vi "Fpga-AXI-Stream.vi"() -> ()   [LabVIEW 2017]
uses:
  <vilib>/Platform/TimedLoop/XDataNode/timing_clust.ctl
  <vilib>/Platform/TimedLoop/XDataNode/nitl_modes.ctl
  <vilib>/Platform/TimedLoop/XDataNode/wakeup.ctl
  <vilib>/rvi/Emulation/niFpgaSctlEmulationGetInTimedLoop.vi
  <vilib>/rvi/Emulation/niFpgaEmulationReportErrorSimple.vi
  <vilib>/rvi/Emulation/niFpgaGetClockAttributes.vi
  <vilib>/rvi/Emulation/niFpgaCriticalErrorInLSC.vi
  <vilib>/rvi/interface/RandomDataEmulation/niFpgaRandomDataHandleErrors.vi
  <vilib>/Platform/TimedLoop/XDataNode/XDataNode.xnode
  <vilib>/rvi/DataTransferAndStorage/Container/XNode/niFpgaContainer.xnode
  <vilib>/rvi/interface/RandomDataEmulation/nirviRandomDataFpgaReadWriteTemplate.vi
  <vilib>/Platform/TimedLoop/XDataNode/XDNodeRunTimeDep.lvlib
  <vilib>/rvi/IPIntegrationNode/IPINode_Typedef/niFpgaIPINodeSupportedFamilies.ctl
  <vilib>/rvi/IPIntegrationNode/IPINode_Utilities/niFpgaIPINodeSimCore.vi
  <vilib>/rvi/IPIntegrationNode/IPINode_Xnode/niFpgaIPINode.xnode
  IP_Block_1SimFiles/xsim.dir/d_microblaze_wrapper_top/xsimkD566ABB023B84B7CB0097135CB091ED7.dll
panel:
  in  "sys_reset":bool
  in  "AXI_STR_RXD_tvalid":bool
  in  "AXI_STR_RXD_tlast":bool
  in  "AXI_STR_RXD_tdata":u32
  in  "AXI_STR_TXD_tready":bool
  out "AXI_STR_RXD_tready":bool
  out "AXI_STR_TXD_tvalid":bool
  out "AXI_STR_TXD_tlast":bool
  out "GPIO2_tri_o":u32
  out "AXI_STR_TXD_tdata":u32
  in  "GPIO1_tri_i":u32
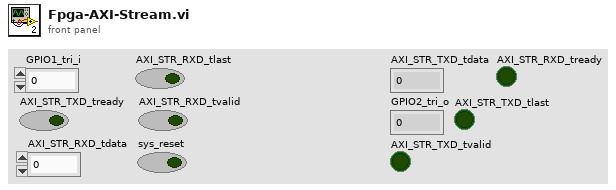
[diagram p1: front panel]
types:
  T1 = typedef "XDNodeRunTimeDep.lvlib/timing_clust.ctl" = cluster{"Expected End [f-1]":u64, "Actual End [f-1]":u64, "Finished Late? [f-1]":bool, "Expected End [i-1]":u64, "Actual End [i-1]":u64, "Finished Late? [i-1]":bool, "Expected Start [i]":u64, "Actual Start [i]":u64, "Expected Start [f]":u64, "Actual Start [f]":u64, "Source Name":string, "Structure Name":string, "Period":i64, "Deadline":i64, "Offset":i64, "Start":i64, "Priority":i32, "Timeout":i32, "Mode":T2, "Wakeup Reason":T3, "Error":errorcluster, "Source Type":string, "Secondary Source Type":string, "Global End Time":u64, "Global Start Time":u64, "Frame Duration":u64, "Iteration Duration":u64, "Assigned CPU":i32, "I/O Scan Engine Mode":u32}
  T2 = typedef "XDNodeRunTimeDep.lvlib/nitl_modes.ctl" = enum32{"No Change", "Process missed periods, maintain original phase", "Discard missed periods, maintain original phase", "Process missed periods, ignore original phase", "Discard missed periods, ignore original phase"}
  T3 = typedef "XDNodeRunTimeDep.lvlib/wakeup.ctl" = enum32{"Normal", "Aborted", "Asynchronous wakeup", "Timing source error", "Timed loop error", "Timeout"}
  T4 = typedef "niFpgaIPINodeSupportedFamilies.ctl" = cluster{"unlimited?":bool, "supported targets":string[]}
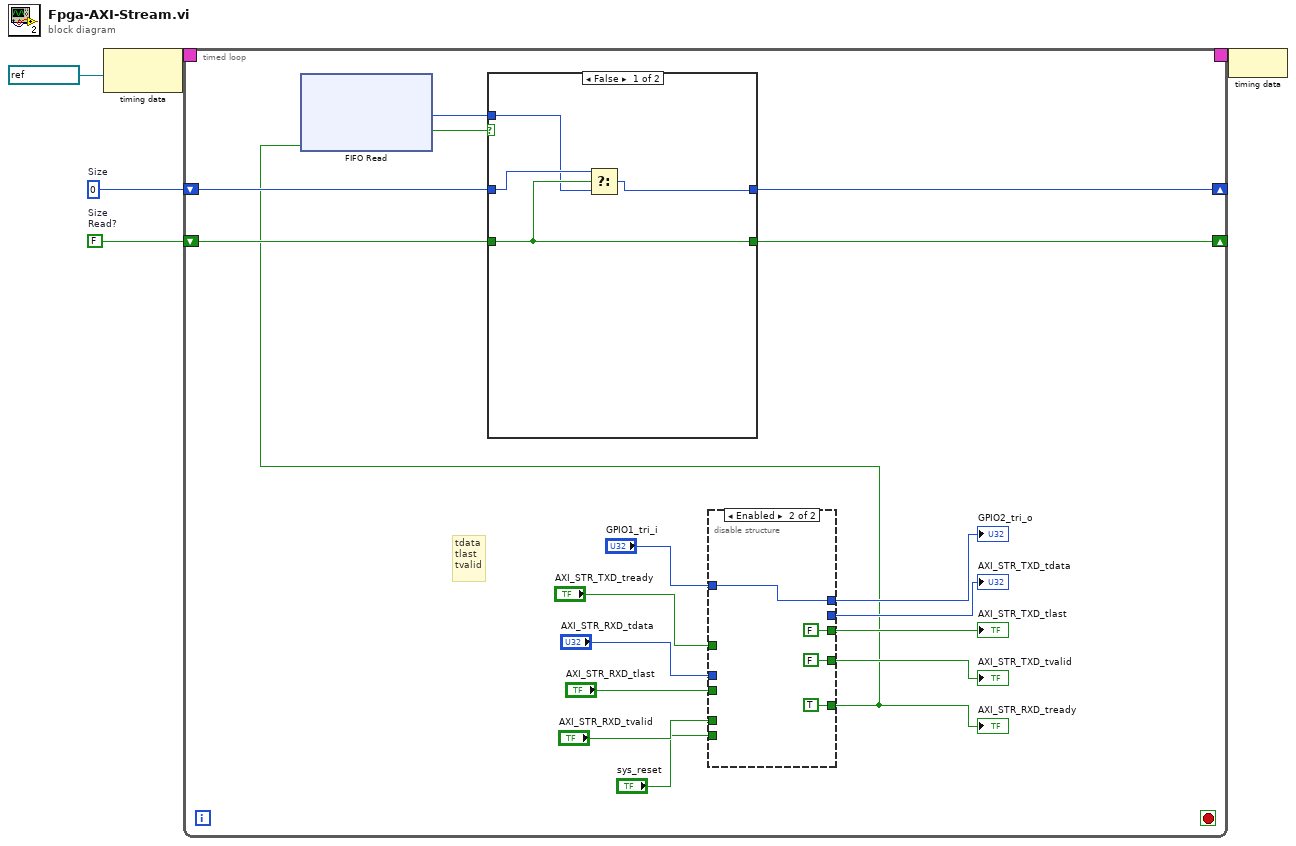
[diagram p0: block diagram]
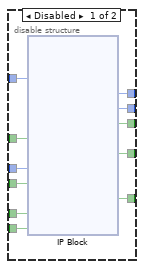
[diagram p2: hidden frame]
diagram:
  w2 = FALSE  # Size Read?
  w1 = u32 0  # Size
  n1 = node-c288(refnum<k21> "100MHz" ("Source Name")) -> (w5:T1)
  n2 = timed-loop {
    timing: w5 -> [_]
    timing-out: [_] -> w4
    shift-right: [w20] -> _
    shift-left: w2 -> [w21]
    shift-right: [w17] -> _
    shift-left: w1 -> [w19]
    stop <- _ stop-if-true
    # "tdata\ntlast\ntvalid"
    n3 = disable-structure shown="Enabled" {
      disable-tunnel: "GPIO1_tri_i" -> [w33 w121]
      disable-tunnel: [w32 _] -> w15
      disable-tunnel: [w31 w121] -> w14
      disable-tunnel: [w30 FALSE ("AXI_STR_TXD_tlast")] -> w13
      disable-tunnel: [w29 FALSE ("AXI_STR_TXD_tvalid")] -> w12
      disable-tunnel: [w28 TRUE ("AXI_STR_RXD_tready")] -> w6
      disable-tunnel: "AXI_STR_TXD_tready" -> [w27 _]
      disable-tunnel: "AXI_STR_RXD_tdata" -> [w26 _]
      disable-tunnel: "AXI_STR_RXD_tlast" -> [w25 _]
      disable-tunnel: "AXI_STR_RXD_tvalid" -> [w24 _]
      disable-tunnel: "sys_reset" -> [w23 _]
      frame Disabled {
        n4 = xnode ("IP Block")("GPIO1_tri_i"=w33, "AXI_STR_TXD_tready"=w27, "AXI_STR_RXD_tdata"=w26, "AXI_STR_RXD_tlast"=w25, "AXI_STR_RXD_tvalid"=w24, "sys_reset"=w23) -> ("GPIO2_tri_o"=w31:u32, "AXI_STR_TXD_tdata"=w32:u32, "AXI_STR_TXD_tlast"=w30:bool, "AXI_STR_TXD_tvalid"=w29:bool, "AXI_STR_RXD_tready"=w28:bool)  [unwired: 1 out]
      }
      frame Enabled {
      }
    }
    "AXI_STR_TXD_tdata" <- w15
    "GPIO2_tri_o" <- w14
    "AXI_STR_TXD_tlast" <- w13
    "AXI_STR_TXD_tvalid" <- w12
    "AXI_STR_RXD_tready" <- w6
    n5 = xnode "FIFO Read"("Ready for Output"=w6) -> ("Element"=w18:u32, "Output Valid"=w22:bool)  [unwired: 1 in, 1 out]
    n6 = case shown="False" w22 {
      tunnel: w21 -> [w125 w126]
      tunnel: [w125 w126] -> w20
      tunnel: w19 -> [w124 w127]
      tunnel: w18 -> [w123 _]
      tunnel: [w122 w127] -> w17
      frame False {
        n7 = Select(t=w124, s=w125, f=w123) -> (s? t:f=w122:u32)
      }
      frame True {
      }
    }
  }
  n8 = node-c288(w4) -> ()
